vi "Main.vi"() -> ()   [LabVIEW 2019]
uses:
  #enum_Language.ctl
  Polish/Polish.lvclass
  C:/Users/Kasia/Desktop/EG COURSES/OOP InProgress/Exercises Workbook/Solutions/Exercise 5/AbstractLanguage/AbstractLanguage.lvclass
  English/English.lvclass
  AbstractLanguage/AbstractLanguage.lvclass
panel:
  out "Error out":errorcluster
  in  "Language":T1
  out "Greeting String":string
  in  "Hello (T)/Goodbye(F)":bool
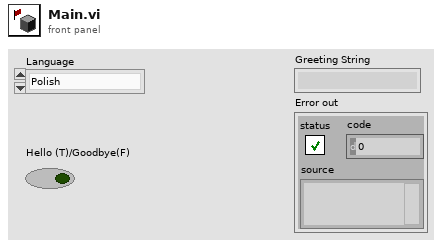
[diagram p1: front panel]
types:
  T1 = typedef "#enum_Language.ctl" = enum16{"Polish", "English"}
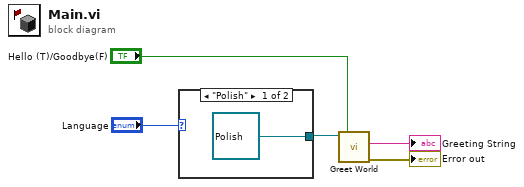
[diagram p0: block diagram]
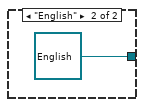
[diagram p2: hidden frame]
diagram:
  n1 = case shown="\"Polish\"" "Language" {
    tunnel: [refnum<class "Polish.lvclass"> refnum ("Polish.lvclass") refnum<class "English.lvclass"> refnum ("English.lvclass")] -> w3
    frame "Polish" {
    }
    frame "English" {
    }
  }
  n2 = call-dynamic "Greet World.vi"("Hello (T)/Goodbye(F)"="Hello (T)/Goodbye(F)", "AbstractLanguage in"=w3) -> ("error out"=→"Error out":errorcluster, "Grreting String"=→"Greeting String":string)  [unwired: 7 in, 1 out]
